vi "Global Refnums.vi"() -> ()   [LabVIEW 2013]
panel:
  out "Reset Shot?":bool
  in  "Setpoint":dbl
  out "Close":bool
  out "Out":bool
  out "In":bool
  out "Compressor boolean":bool
  out "Far":bool
  in  "Actual":dbl
  out "Tension":bool
  out "Gyro":string
  out "Run Rollermotor in Auton":bool
  in  "Shoot angle":dbl
  out "Fire":bool
  out "Arm":string
  out "Winch":string
  in  "Counter BR":string
  in  "Counter BL":string
  in  "Counter FR":string
  in  "Counter FL":string
  in  "Counter BR (rate)":dbl
  in  "Counter FR (rate)":dbl
  in  "Counter BL (rate)":dbl
  in  "Counter FL (rate)":dbl
  in  "Counter BR (distance)":dbl
  in  "Counter FR (distance)":dbl
  in  "Counter BL (distance)":dbl
  in  "Counter FL (distance)":dbl
  out "Ball stop up":string
  out "Ball clamp out":string
  out "Floor Pick-Up":string
  out "Shooter Angle":string
  out "Shooter Winch Latch":string
  out "Compressor":string
  out "RollerMotor":string
  out "Joystick R 1":string
  out "WinchMotor":string
  out "LoadCell":string
  out "Joystick L 1":string
  out "Rotational Motor BL":string
  out "Rotational Motor BR":string
  out "Rotational Motor FL":string
  out "Rotational Motor FR":string
  out "Drive Motor BL":string
  out "Drive Motor BR":string
  out "Drive Motor FL":string
  out "Drive Motor FR":string
  out "V Encoder BL":string
  out "V Encoder BR":string
  out "V Encoder FL":string
  out "V Encoder FR":string
  out "A Encoder BL":string
  out "A Encoder BR":string
  out "A Encoder FL":string
  out "A Encoder FR":string
  # "Encoders"
  # "Motors"
  # "Joysticks"
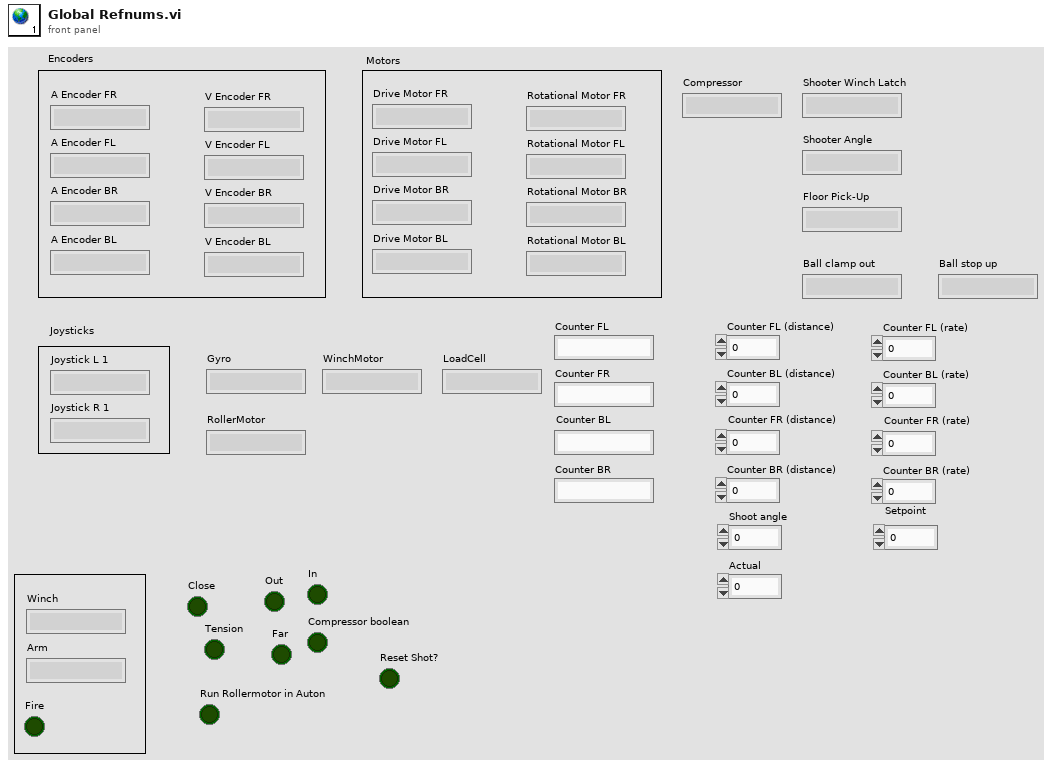
[diagram p1: front panel]
diagram:
